vi "Update PV.vi"(8 "error in (no error)":errorcluster, 10 "PV":refnum<class "PV.lvclass">, 11 "CS++FgenGui in":refnum<class "CS++FgenGui.lvclass">) -> (0 "error out":errorcluster, 3 "CS++FgenGui out":refnum<class "CS++FgenGui.lvclass">)   [LabVIEW 2013, in "CS++FgenGui.lvlib" / "CS++FgenGui.lvclass"]
doc: "Update value of PV on GUI via event."
uses:
  CS++FgenGui.lvclass
  Core/Classes/CS++ProcessVariables/ProcessVariable/PV.lvclass
  CS++FgenGui.lvclass/CS++FgenGui.ctl
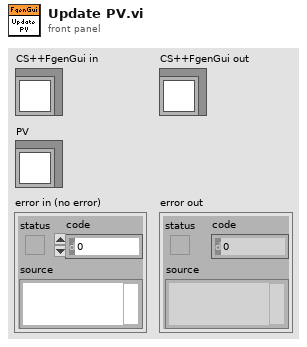
[diagram p1: front panel]
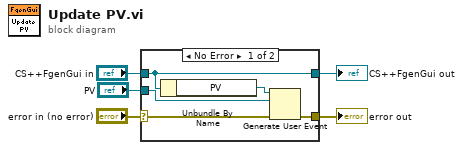
[diagram p0: block diagram]
diagram:
  n1 = case shown="No Error" "error in (no error)" {
    selector: "error in (no error)" -> [w7 w12]
    tunnel: [w6 w12] -> w3
    tunnel: [w10 w11] -> w4
    tunnel: "CS++FgenGui in" -> [w10 w11]
    tunnel: "PV" -> [w8 _]
    frame No Error {
      n2 = Unbundle By Name(w10) -> ("PV"=w9:refnum<user-event>)
      n3 = Generate User Event(user event=w9, event data cluster=w8, error in=w7) -> (error out=w6:errorcluster)  [unwired: 1 in, 1 out]
    }
    frame Error {
    }
  }
  "error out" <- w3
  "CS++FgenGui out" <- w4
